vi "Parse Frame Config Data(SubVI).vi"(8 "error in (no error)":errorcluster, 11 "all rows":string[][](array[string])) -> (0 "error out":errorcluster, 3 "Data Array out":T1[](array[typedef]) {"Data" format="%x"; "Start_Addr" format="%x"})   [LabVIEW 2018, in "Config_Read_BML.lvclass"]
uses:
  Config_Read_BML.lvclass
  Frame_Data.ctl
  OperationMode.ctl
  BurstLength.ctl
  RW_Option.ctl
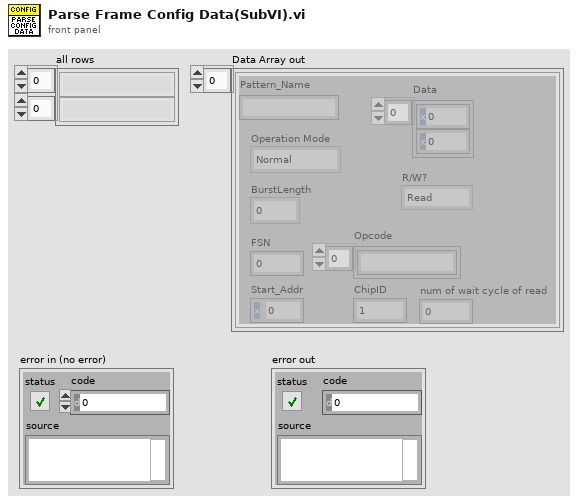
[diagram p1: front panel]
types:
  T1 = typedef "Config_Read_BML.lvclass/Frame_Data.ctl" = cluster{"Pattern_Name":string, "Operation Mode":T2, "BurstLength":T3, "FSN":u8, "Start_Addr":u16, "Data":u8[], "R/W?":T4, "Opcode":string[], "ChipID":u8, "num of wait cycle of read":i8}
  T2 = typedef "Config_Read_BML.lvclass/OperationMode.ctl" = enum8{"Normal", "ImmeEffect", "InitSlaveID", "LoadData"}
  T3 = typedef "Config_Read_BML.lvclass/BurstLength.ctl" = enum8{"0", "2", "3", "4", "5", "8", "16", "32"}
  T4 = typedef "Config_Read_BML.lvclass/RW_Option.ctl" = enum16{"Read", "Write", "R/W"}
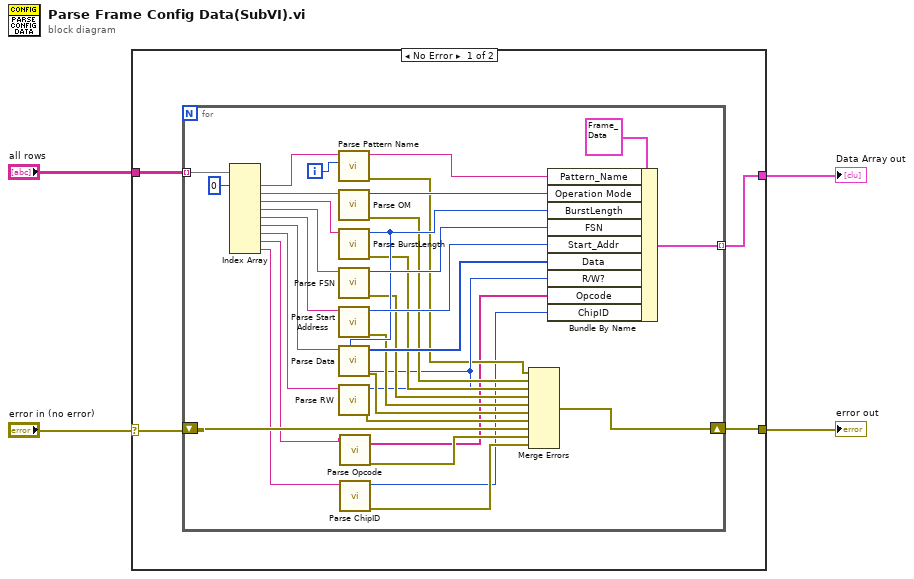
[diagram p0: block diagram]
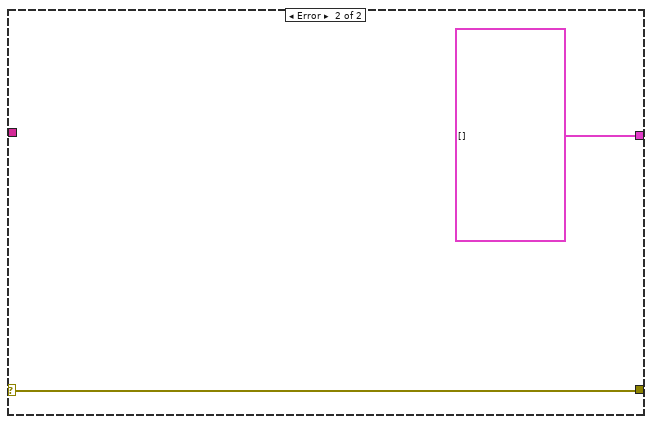
[diagram p2: hidden frame]
diagram:
  n1 = case shown="No Error" "error in (no error)" {
    selector: "error in (no error)" -> [w7 w44]
    tunnel: "all rows" -> [w8 _]
    tunnel: [w6 w44] -> w2
    tunnel: [w5 T1[] []] -> w1
    frame No Error {
      n2 = for {
        tunnel: w8 -> [w42] mode=indexing
        shift-right: [w21] -> w6
        shift-left: w7 -> [w22]
        tunnel: [w20] -> w5 mode=indexing
        i -> [w17]
        n3 = Index Array(array=w42, index #1=0 ("index")) -> (element #1=w18:string, element #2=w39:string, element #3=w37:string, element #4=w36:string, element #5=w34:string, element #6=w32:string, element #7=w29:string, element #8=w14:string, element #9=w11:string)  [unwired: 8 in]
        n4 = call "Parse Pattern Name.vi"("Index"=w17, "Pattern Name"=w18) -> ("error out"=w16:errorcluster, "Pattern Name out"=w15:string)  [unwired: 8 in]
        n5 = call "Parse OM.vi"("OM in"=w39) -> ("error out"=w28:errorcluster, "OM out"=w38:T2)  [unwired: 9 in]
        n6 = call "Parse BurstLength.vi"("Burst Length in"=w37) -> ("error out"=w27:errorcluster, "BurstLength Out"=w31:T3)  [unwired: 9 in]
        n7 = call "Parse FSN.vi"("FSN in"=w36) -> ("error out"=w26:errorcluster, "FSN out"=w35:u8)  [unwired: 9 in]
        n8 = call "Parse Start Address.vi"("Addr in"=w34) -> ("error out"=w25:errorcluster, "Addr out"=w33:u16)  [unwired: 9 in]
        n9 = call "Parse RW.vi"("R/W mode in"=w29) -> ("error out"=w23:errorcluster, "R/W?"=w19:T4)  [unwired: 9 in]
        n10 = call "Parse Data.vi"("R/W?"=w19, "BurstLength"=w31, "Data in"=w32) -> ("error out"=w24:errorcluster, "Data Array out"=w30:u8[])  [unwired: 7 in]
        n11 = call "Parse Opcode.vi"("Opcode"=w14) -> ("Error out"=w13:errorcluster, "Opcode Array"=w12:string[])  [unwired: 9 in]
        n12 = call "Parse ChipID.vi"("String"=w11) -> ("error out"=w10:errorcluster, "ChipID"=w9:u8)  [unwired: 9 in]
        n13 = Merge Errors(w16, w28, w27, w26, w25, w24, w23, w22, w13, w10) -> (w21:errorcluster)
        n14 = Bundle By Name(cluster=T1 {"Pattern_Name"="", "Operation Mode"=enum."Normal", "BurstLength"=enum."0", "FSN"=0, "Start_Addr"=0, "Data"=[], "R/W?"=enum."Read", "Opcode"=[], "ChipID"=1, "num of wait cycle of read"=0} ("Frame_Data"), "Pattern_Name"=w15, "Operation Mode"=w38, "BurstLength"=w31, "FSN"=w35, "Start_Addr"=w33, "Data"=w30, "R/W?"=w19, "Opcode"=w12, "ChipID"=w9) -> (w20:T1)
      }
    }
    frame Error {
    }
  }
  "error out" <- w2
  "Data Array out" <- w1
